vi "Voltages.vi"(11 "file path (dialog if empty)":path) -> ()   [LabVIEW 2014]
uses:
  <vilib>/Utility/file.llb/Write To Spreadsheet File (DBL).vi
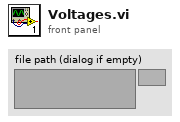
[diagram p1: front panel]
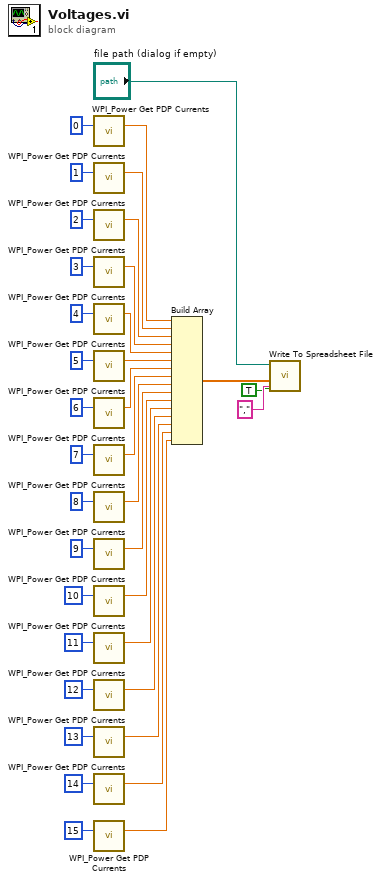
[diagram p0: block diagram]
diagram:
  n1 = call <vilib>:"WPI_Power Get PDP Currents.vi"("PDP Channel"=0) -> ("current (A)"=w33:dbl)  [unwired: 12 in, 2 out]
  n2 = call <vilib>:"WPI_Power Get PDP Currents.vi"("PDP Channel"=1) -> ("current (A)"=w31:dbl)  [unwired: 12 in, 2 out]
  n3 = call <vilib>:"WPI_Power Get PDP Currents.vi"("PDP Channel"=2) -> ("current (A)"=w29:dbl)  [unwired: 12 in, 2 out]
  n4 = call <vilib>:"WPI_Power Get PDP Currents.vi"("PDP Channel"=3) -> ("current (A)"=w27:dbl)  [unwired: 12 in, 2 out]
  n5 = call <vilib>:"WPI_Power Get PDP Currents.vi"("PDP Channel"=4) -> ("current (A)"=w25:dbl)  [unwired: 12 in, 2 out]
  n6 = call <vilib>:"WPI_Power Get PDP Currents.vi"("PDP Channel"=5) -> ("current (A)"=w23:dbl)  [unwired: 12 in, 2 out]
  n7 = call <vilib>:"WPI_Power Get PDP Currents.vi"("PDP Channel"=6) -> ("current (A)"=w21:dbl)  [unwired: 12 in, 2 out]
  n8 = call <vilib>:"WPI_Power Get PDP Currents.vi"("PDP Channel"=7) -> ("current (A)"=w19:dbl)  [unwired: 12 in, 2 out]
  n9 = call <vilib>:"WPI_Power Get PDP Currents.vi"("PDP Channel"=8) -> ("current (A)"=w17:dbl)  [unwired: 12 in, 2 out]
  n10 = call <vilib>:"WPI_Power Get PDP Currents.vi"("PDP Channel"=9) -> ("current (A)"=w15:dbl)  [unwired: 12 in, 2 out]
  n11 = call <vilib>:"WPI_Power Get PDP Currents.vi"("PDP Channel"=10) -> ("current (A)"=w13:dbl)  [unwired: 12 in, 2 out]
  n12 = call <vilib>:"WPI_Power Get PDP Currents.vi"("PDP Channel"=11) -> ("current (A)"=w11:dbl)  [unwired: 12 in, 2 out]
  n13 = call <vilib>:"WPI_Power Get PDP Currents.vi"("PDP Channel"=12) -> ("current (A)"=w9:dbl)  [unwired: 12 in, 2 out]
  n14 = call <vilib>:"WPI_Power Get PDP Currents.vi"("PDP Channel"=13) -> ("current (A)"=w6:dbl)  [unwired: 12 in, 2 out]
  n15 = call <vilib>:"WPI_Power Get PDP Currents.vi"("PDP Channel"=14) -> ("current (A)"=w5:dbl)  [unwired: 12 in, 2 out]
  n16 = call <vilib>:"WPI_Power Get PDP Currents.vi"("PDP Channel"=15) -> ("current (A)"=w3:dbl)  [unwired: 12 in, 2 out]
  n17 = Build Array(w33, w31, w29, w27, w25, w23, w21, w19, w17, w15, w13, w11, w9, w6, w5, w3) -> (w1:dbl[])
  n18 = call-poly <vilib>:"Write To Spreadsheet File.vi"("delimiter (\\t)"="," ("delimiter (\\t)"), "append to file? (new file:F)"=TRUE, "1D data"=w1, "file path (dialog if empty)"="file path (dialog if empty)") -> ()  [unwired: 4 in, 1 out]
